vi "calc_temp_masses.vi"(0 "Cell Temps (uncorr)":dbl[](array[numeric]), 1 "Total HCl Volumes (uncorr)":dbl[](array[numeric]), 5 "HCl Temp (burret)":dbl, 7 "Salinity":dbl, 9 "Sample Size":dbl, 11 "Sample Units":bool, 12 "Sample Temp (uncorr)":dbl, 13 "Alkalinity Calculation Functions":T1) -> (4 "Corrected HCl Volumes":dbl[](array[numeric]), 6 "Total HCl masses":dbl[](array[numeric]), 8 "Corrected Cell Temperature Mean":dbl format="%.2f", 10 "Sample Mass":dbl, 15 "k":dbl)   [LabVIEW 2010]
uses:
  <vilib>/gmath/NI_Gmath.lvlib
  <vilib>/Analysis/NI_AALBase.lvlib
panel:
  out "HCl Density":dbl format="%.2f"
  out "Corrected HCl Temperature":dbl format="%.2f"
  out "Corrected Sample Temperature":dbl format="%.2f"
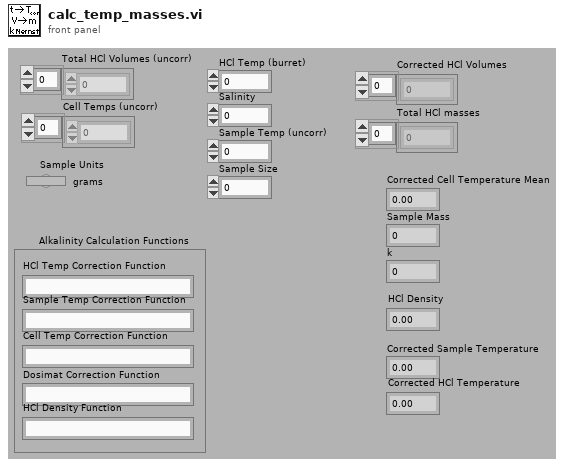
[diagram p1: front panel]
types:
  T1 = cluster{"HCl Temp Correction Function":string, "Sample Temp Correction Function":string, "Dosimat Correction Function":string, "Cell Temp Correction Function":string, "HCl Density Function":string}
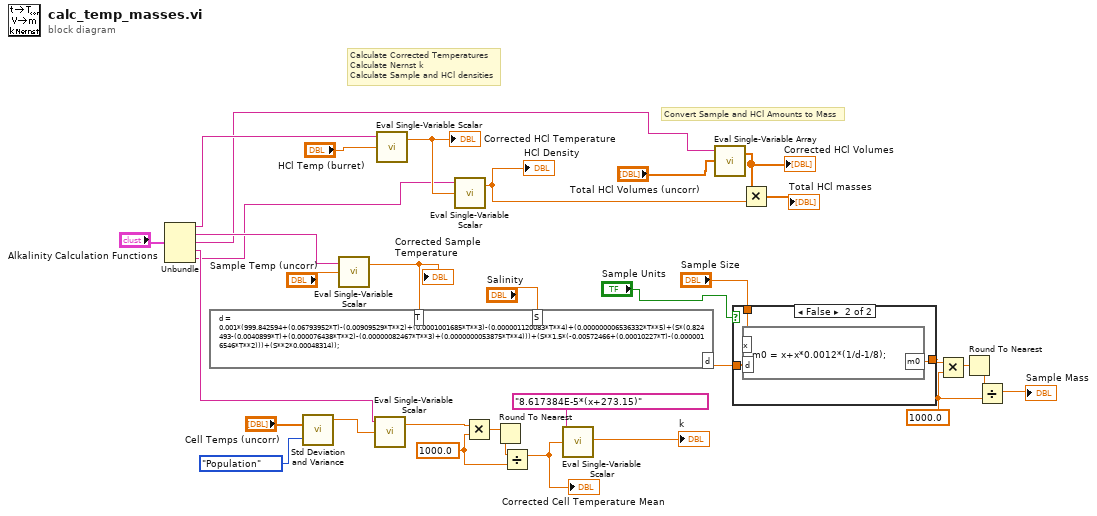
[diagram p0: block diagram]
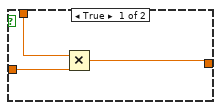
[diagram p2: hidden frame]
diagram:
  w23 = 1000.0 ("y")
  w27 = 1000.0 ("y")
  # "Convert Sample and HCl Amounts to Mass"
  # "Calculate Corrected Temperatures\nCalculate Nernst k\nCalculate Sample and HCl densities"
  n1 = Unbundle("Alkalinity Calculation Functions") -> ("HCl Temp Correction Function"=w13:string, "Sample Temp Correction Function"=w12:string, "Dosimat Correction Function"=w11:string, "Cell Temp Correction Function"=w10:string, "HCl Density Function"=w9:string)
  n2 = call <vilib>:"Std Deviation and Variance.vi"("X"="Cell Temps (uncorr)", "Weighting (Sample)"=enum16{"Sample", "Population"}."Population") -> ("mean"=w21:dbl)  [unwired: 2 out]
  n3 = call <vilib>:"Eval Single-Variable Scalar.vi"("x value"="Sample Temp (uncorr)", "formula"=w12) -> ("y value"=w19:dbl)  [unwired: 1 in, 1 out]
  "Corrected Sample Temperature" <- w19
  n4 = formula code="d = 0.001*(999.842594+(0.06793952*T)-(0.00909529*T**2)+(0.0001001685*T**3)-(0.000001120083*T**4)+(0.000000006536332*T**5)+(S*(0.824493-(0.0040899*T)+(0.000076438*T**2)-(0.00000082467*T**3)+(0.0000000053875*T**4)))+(S**1.5*(-0.00572466+(0.00010227*T)-(0.0000016546*T**2)))+(S**2*0.00048314));"("T"=w19, "S"="Salinity") -> ("d"=w29:dbl)
  n5 = call <vilib>:"Eval Single-Variable Scalar.vi"("x value"=w21, "formula"=w10) -> ("y value"=w22:dbl)  [unwired: 1 in, 1 out]
  n6 = call <vilib>:"Eval Single-Variable Scalar.vi"("x value"="HCl Temp (burret)", "formula"=w13) -> ("y value"=w31:dbl)  [unwired: 1 in, 1 out]
  "Corrected HCl Temperature" <- w31
  n7 = call <vilib>:"Eval Single-Variable Scalar.vi"("x value"=w31, "formula"=w9) -> ("y value"=w30:dbl)  [unwired: 1 in, 1 out]
  "HCl Density" <- w30
  n8 = Multiply(x=w22, y=w27) -> (x*y=w28:dbl)
  n9 = Round To Nearest(number=w28) -> ()  [unwired: 1 out]
  n10 = Divide(x=w28, y=w27) -> (x/y=w20:dbl)
  "Corrected Cell Temperature Mean" <- w20
  n11 = call <vilib>:"Eval Single-Variable Scalar.vi"("x value"=w20, "formula"="8.617384E-5*(x+273.15)") -> ("y value"=→"k":dbl)  [unwired: 1 in, 1 out]
  n12 = call <vilib>:"Eval Single-Variable Array.vi"("X Values"="Total HCl Volumes (uncorr)", "formula"=w11) -> ("Y Values"=w17:dbl[])  [unwired: 1 in, 1 out]
  "Corrected HCl Volumes" <- w17
  n13 = case "Case" shown="False" "Sample Units" {
    tunnel: w29 -> [w34 w38]
    tunnel: "Sample Size" -> [w35 w37]
    tunnel: [w33 w36] -> w26
    frame True {
      n14 = Multiply(x=w35, y=w34) -> (x*y=w33:dbl)
    }
    frame False {
      n15 = formula code="m0 = x+x*0.0012*(1/d-1/8);"("x"=w37, "d"=w38) -> ("m0"=w36:dbl)
    }
  }
  n16 = Multiply(x=w17, y=w30) -> (x*y=→"Total HCl masses":dbl[])
  n17 = Multiply(x=w26, y=w23) -> (x*y=w25:dbl)
  n18 = Round To Nearest(number=w25) -> (nearest integer value=w24:dbl)
  n19 = Divide(x=w24, y=w23) -> (x/y=→"Sample Mass":dbl)
